vi "Actual Replot.vi"(8 "error in (no error)":errorcluster, 11 "XY WFRM Plot in":refnum<class "XY WFRM Plot.lvclass">) -> (0 "error out":errorcluster, 3 "XY WFRM Plot out":refnum<class "XY WFRM Plot.lvclass">)   [LabVIEW 2021, in "XY WFRM Plot.lvclass"]
uses:
  XY WFRM Plot.lvclass
  C:/GitHub/LabActor/Plots/Plot/Plot.lvclass
  Plot/Plot.lvclass/Plot.ctl
  XY WFRM Plot.lvclass/XY WFRM Plot.ctl
  8cb32180-7abd-4b27-afcb-bbd739cf6f07.vi
  e6847e96-357f-421f-be23-6c38e145b2ce.vi
  1432e590-7574-4fdc-991b-60627a69a38a.vi
  c5e1e698-5171-48f6-a2a7-0a8aaa819dda.vi
  372697b9-8762-4fc7-8ff0-8d62db81c817.vi
  27d2bad1-82f0-4063-802e-88bb5171f6f1.vi
  a4261e9a-a62c-4d5f-83e9-7bb19e5e27b0.vi
  Plot/Read Files.vi
  8cb32180-7abd-4b27-afcb-bbd739cf6f07.vi/668a06be-d8be-4049-82ee-33f1cdaacdc4.vi
  8cb32180-7abd-4b27-afcb-bbd739cf6f07.vi/2c6de516-1d23-4c23-bfc5-564dc8149620.vi
  e6847e96-357f-421f-be23-6c38e145b2ce.vi/0532bd49-aff3-45ad-9cc0-a13f982e0e17.vi
  e6847e96-357f-421f-be23-6c38e145b2ce.vi/724fb671-963e-4042-b130-e72c76e88fd9.vi
  <vilib>/Utility/error.llb/Clear Errors.vi
  372697b9-8762-4fc7-8ff0-8d62db81c817.vi/c0c8f4eb-f5dc-43a3-9fd2-6fe82153b517.vi
  372697b9-8762-4fc7-8ff0-8d62db81c817.vi/d9f28dd1-57bc-437c-abf9-381ead6ef493.vi
  8cb32180-7abd-4b27-afcb-bbd739cf6f07.vi/668a06be-d8be-4049-82ee-33f1cdaacdc4.vi/f32759e9-418f-4dd9-99d9-892840a9754a.vi
  e6847e96-357f-421f-be23-6c38e145b2ce.vi/0532bd49-aff3-45ad-9cc0-a13f982e0e17.vi/1bcf6eca-5e38-4694-9c6b-5dcad1ef6d61.vi
  372697b9-8762-4fc7-8ff0-8d62db81c817.vi/c0c8f4eb-f5dc-43a3-9fd2-6fe82153b517.vi/579b74a7-738b-41b6-a2c9-a5c73b95a491.vi
  NHMFL_Core/Libraries/File/TDMS/TDMS Open Err Check.vi
  NHMFL_Core/Libraries/File/Get TDMS channel info.vi
  <vilib>/measure/maresamp.llb/Resample Waveforms (single shot).vi
  <vilib>/measure/maresamp.llb/Resample Waveform (single shot).vi
  NHMFL_Core/Libraries/Utilities/Waveform/AvrgDecimate.vi
  NHMFL_Core/Libraries/Utilities/Waveform/MaxMinDecimate.vi
  Plot/Plot.lvclass
  <vilib>/ErrorRing/Error Ring.xnode
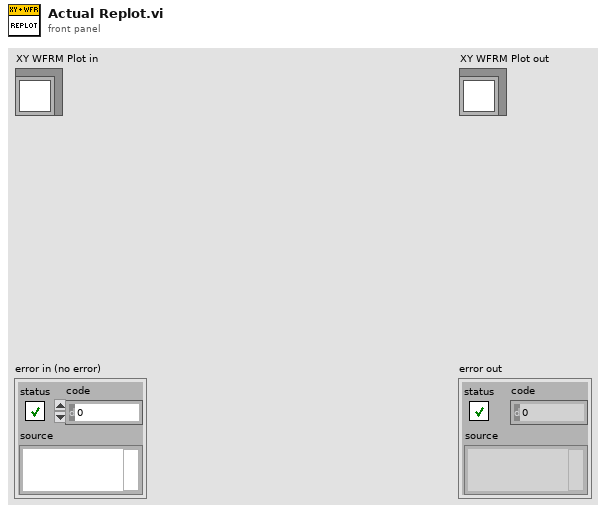
[diagram p1: front panel]
types:
  T1 = typedef "Plot types.ctl" = enum16{"Waveform Plot", "XY Plot", "Full XY"}
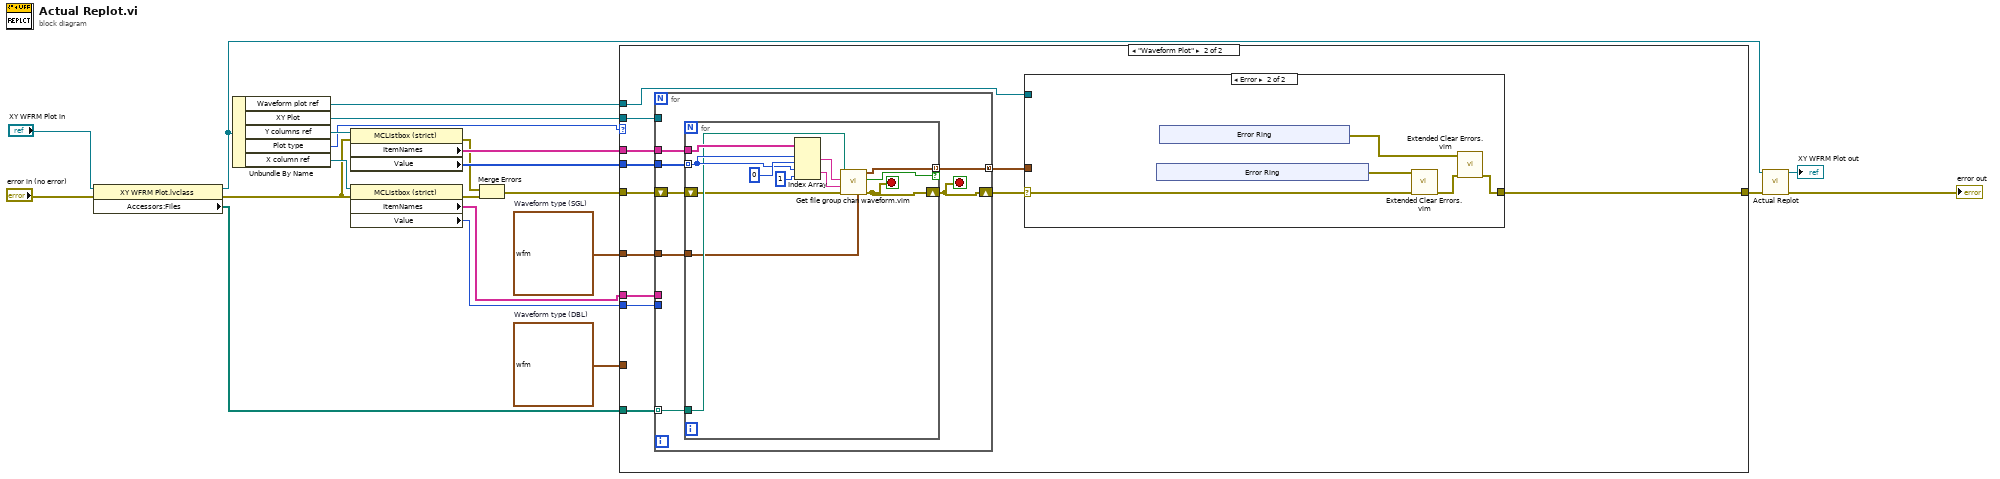
[diagram p0: block diagram]
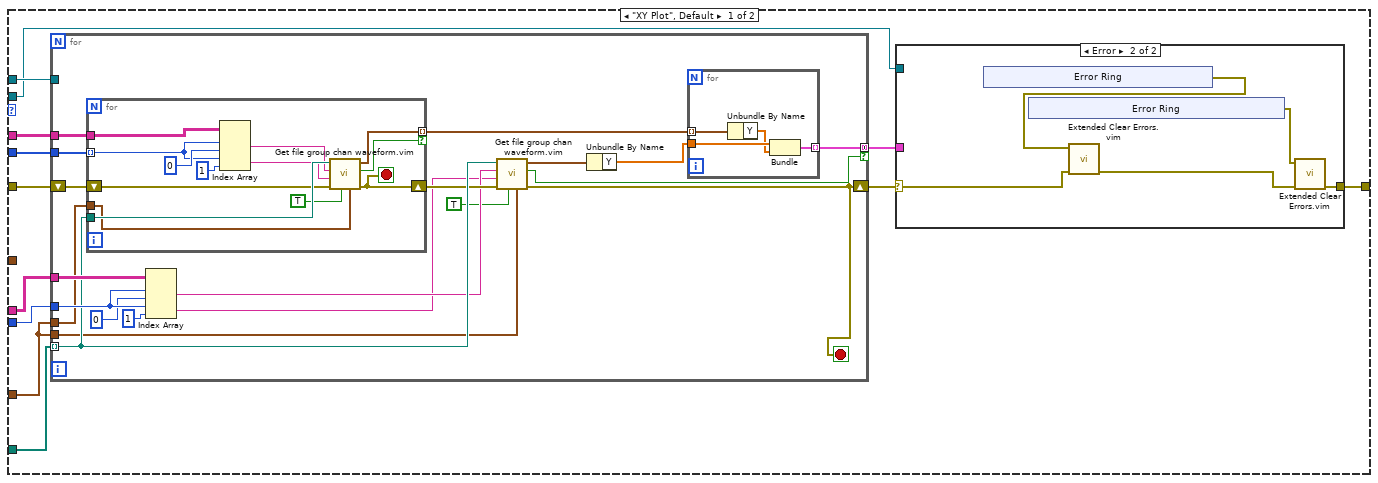
[diagram p2: hidden frame]
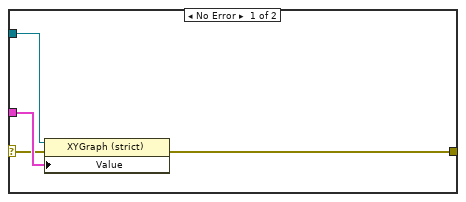
[diagram p3: hidden frame]
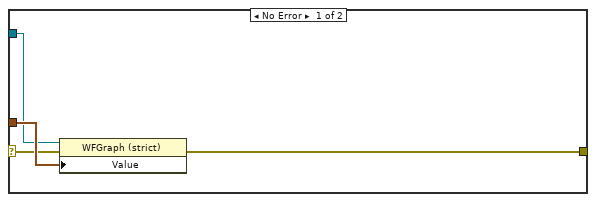
[diagram p4: hidden frame]
diagram:
  w2 = waveform(sgl) {"t0"=timestamp(0 s since 1904-01-01), "dt"=1.0, "Y"=[]}  # Waveform type (SGL)
  w3 = waveform(dbl) {"t0"=timestamp(0 s since 1904-01-01), "dt"=1.0, "Y"=[]}  # Waveform type (DBL)
  n1 = property class="XY WFRM Plot.lvclass"(reference="XY WFRM Plot in", error in="error in (no error)") -> (reference out=w5:refnum<class "XY WFRM Plot.lvclass">, error out=w11:errorcluster, "Accessors:Files"=w18:path[])
  n2 = Unbundle By Name(w5) -> ("Waveform plot ref"=w13:refnum<vi>, "XY Plot"=w14:refnum<vi>, "Y columns ref"=w21:refnum<vi>, "Plot type"=w10:T1, "X column ref"=w17:refnum<vi>)
  n3 = property class="MCListbox (strict)"(reference=w21, error in=w11) -> (error out=w9:errorcluster, "ItemNames"=w20:string[][], "Value"=w19:i32[])  [unwired: 1 out]
  n4 = property class="MCListbox (strict)"(reference=w17, error in=w11) -> (error out=w8:errorcluster, "ItemNames"=w15:string[][], "Value"=w16:i32)  [unwired: 1 out]
  n5 = Merge Errors(w9, w8) -> (w7:errorcluster)
  n6 = case shown="\"Waveform Plot\"" w10 {
    tunnel: w20 -> [w34 w94]
    tunnel: w19 -> [w33 w93]
    tunnel: w18 -> [w32 w92]
    tunnel: w16 -> [w31 w91]
    tunnel: w15 -> [w30 w90]
    tunnel: w14 -> [w26 w89]
    tunnel: w13 -> [w29 w86]
    tunnel: [w27 w87] -> w6
    tunnel: w7 -> [w25 w85]
    tunnel: w3 -> [w23 _]
    tunnel: w2 -> [_ w83]
    frame "XY Plot", Default {
      n7 = for {
        tunnel: w34 -> [w65]
        tunnel: w33 -> [w64]
        tunnel: w32 -> [w60] mode=indexing
        shift-right: [w46] -> w24
        shift-left: w25 -> [w63]
        tunnel: w31 -> [w62]
        tunnel: w30 -> [w61]
        tunnel: w29 -> [_]
        tunnel: [w51] -> w28 mode=concatenating if=w50
        tunnel: w23 -> [w48]
        tunnel: w23 -> [w47]
        stop <- w46 stop-if-true
        n8 = for {
          tunnel: w65 -> [w82]
          tunnel: w64 -> [w80] mode=indexing
          tunnel: w60 -> [w78]
          shift-right: [w71] -> w58
          shift-left: w63 -> [w75]
          tunnel: [w74] -> w59 mode=indexing if=w73
          tunnel: w47 -> [w70]
          stop <- w71 stop-if-true
          n9 = Index Array(array=w82, index (row) #1=w80, index (col) #1=0 ("disabled index (col)"), index (row) #2=w80, index (col) #2=1 ("disabled index (col)")) -> (element #1=w77:string, element #2=w76:string)
          n10 = call "Get file group chan waveform.vim"("Waveform type"=w70, "Clear missing ch err"=TRUE, "Error In"=w75, "Channel"=w76, "Group"=w77, "File"=w78) -> ("Error Out"=w71:errorcluster, "Valid WFRM"=w73:bool, "Waveform"=w74:waveform(dbl))  [unwired: 3 in]
        }
        n11 = Index Array(array=w61, index (row) #1=w62, index (col) #1=0 ("index (col)"), index (row) #2=w62, index (col) #2=1 ("index (col)")) -> (element #1=w55:string, element #2=w54:string)
        n12 = call "Get file group chan waveform.vim"("Waveform type"=w48, "Clear missing ch err"=TRUE, "Error In"=w58, "Channel"=w54, "Group"=w55, "File"=w60) -> ("Error Out"=w46:errorcluster, "Valid WFRM"=w50:bool, "Waveform"=w53:waveform(dbl))  [unwired: 3 in]
        n13 = Unbundle By Name(w53) -> ("Y"=w52:dbl[])
        n14 = for {
          tunnel: w52 -> [w69]
          tunnel: w59 -> [w68] mode=indexing
          tunnel: [w66] -> w51 mode=indexing
          n15 = Unbundle By Name(w68) -> ("Y"=w67:dbl[])
          n16 = Bundle("Y"=w69, "Y"=w67) -> (w66:cluster{"Y":dbl[], "Y":dbl[]})  [unwired: 1 in]
        }
      }
      n17 = case shown="Error" w24 {
        selector: w24 -> [w35 w41]
        tunnel: w28 -> [w38 _]
        tunnel: [w37 w42] -> w27
        tunnel: w26 -> [w36 _]
        frame No Error {
          n18 = property class="XYGraph (strict)"(reference=w36, error in=w35, "Value"=w38) -> (error out=w37:errorcluster)  [unwired: 1 out]
        }
        frame Error {
          n19 = xnode "Error Ring"() -> ("error out"=w39:errorcluster)
          n20 = xnode "Error Ring"() -> ("error out"=w43:errorcluster)
          n21 = call "Extended Clear Errors.vim"("Error In"=w41, "specific error code to clear (0: all)"=w39) -> ("Error Out"=w40:errorcluster)  [unwired: 7 in, 2 out]
          n22 = call "Extended Clear Errors.vim"("Error In"=w40, "specific error code to clear (0: all)"=w43) -> ("Error Out"=w42:errorcluster)  [unwired: 7 in, 2 out]
        }
      }
    }
    frame "Waveform Plot" {
      n23 = for {
        tunnel: w94 -> [w112]
        tunnel: w93 -> [w111]
        tunnel: w92 -> [w109] mode=indexing
        shift-right: [w107] -> w84
        shift-left: w85 -> [w110]
        tunnel: w91 -> [_]
        tunnel: w90 -> [_]
        tunnel: w89 -> [_]
        tunnel: [w108] -> w88 mode=concatenating
        tunnel: w83 -> [w106]
        stop <- w107 stop-if-true
        n24 = for {
          tunnel: w112 -> [w124]
          tunnel: w111 -> [w122] mode=indexing
          tunnel: w109 -> [w120]
          shift-right: [w114] -> w107
          shift-left: w110 -> [w117]
          tunnel: [w116] -> w108 mode=indexing if=w115
          tunnel: w106 -> [w113]
          stop <- w114 stop-if-true
          n25 = Index Array(array=w124, index (row) #1=w122, index (col) #1=0 ("disabled index (col)"), index (row) #2=w122, index (col) #2=1 ("disabled index (col)")) -> (element #1=w119:string, element #2=w118:string)
          n26 = call "Get file group chan waveform.vim"("Waveform type"=w113, "Error In"=w117, "Channel"=w118, "Group"=w119, "File"=w120) -> ("Error Out"=w114:errorcluster, "Valid WFRM"=w115:bool, "Waveform"=w116:waveform(sgl))  [unwired: 4 in]
        }
      }
      n27 = case shown="Error" w84 {
        selector: w84 -> [w95 w103]
        tunnel: w88 -> [w98 _]
        tunnel: [w97 w100] -> w87
        tunnel: w86 -> [w96 _]
        frame No Error {
          n28 = property class="WFGraph (strict)"(reference=w96, error in=w95, "Value"=w98) -> (error out=w97:errorcluster)  [unwired: 1 out]
        }
        frame Error {
          n29 = xnode "Error Ring"() -> ("error out"=w102:errorcluster)
          n30 = xnode "Error Ring"() -> ("error out"=w99:errorcluster)
          n31 = call "Extended Clear Errors.vim"("Error In"=w103, "specific error code to clear (0: all)"=w102) -> ("Error Out"=w101:errorcluster)  [unwired: 7 in, 2 out]
          n32 = call "Extended Clear Errors.vim"("Error In"=w101, "specific error code to clear (0: all)"=w99) -> ("Error Out"=w100:errorcluster)  [unwired: 7 in, 2 out]
        }
      }
    }
  }
  n33 = call-parent "Actual Replot.vi"("error in (no error)"=w6, "Plot in"=w5) -> ("error out"=→"error out":errorcluster, "Plot out"=→"XY WFRM Plot out":refnum<class "XY WFRM Plot.lvclass">)  [unwired: 8 in]
